vi "IMAQ FPGA Camera Link Pixel Packer U16x1.vi"(8 "Input Valid":bool, 9 "Frame Valid In":bool, 10 "Line Valid In":bool, 11 "Pixel In":u16) -> (0 "Output Valid":bool, 1 "Frame Valid Out":bool, 2 "Line Valid Out":bool, 3 "Pixel Bus x8 Out":cluster{"Pixels":u16[], "DV":bool[]})   [LabVIEW 2020]
doc: "The Pixel Packer combines pixels from different cycles to create a Pixel Bus with 8 adjacent pixels. The DV flag in the Pixel Bus x8 Out indicates if the corresponding pixel is valid in case there are cameras with a width that is not a multiple of 8."
uses:
  <vilib>/visionFPGA/Basics/Camera Link Acquisition/Controls/IMAQ FPGA Camera Link Pixel Packer State.ctl
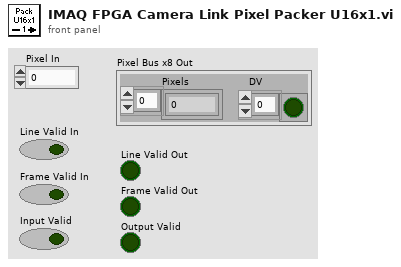
[diagram p1: front panel]
types:
  T1 = typedef "IMAQ FPGA Camera Link Pixel Packer State.ctl" = enum16{"Wait to Pack", "Pack", "Add EOL", "Check EOI"}
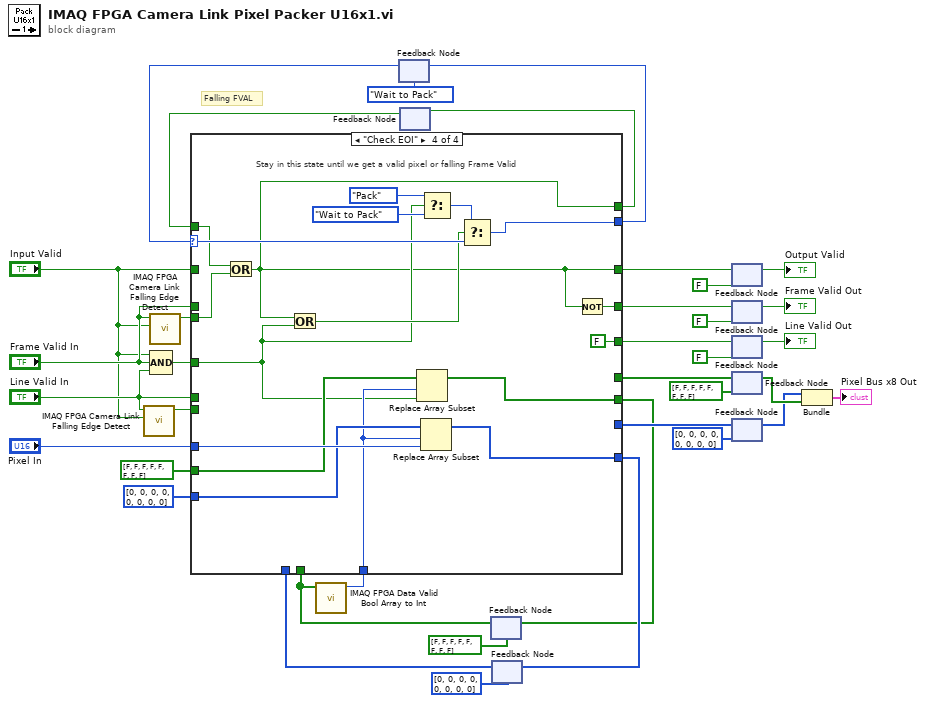
[diagram p0: block diagram]
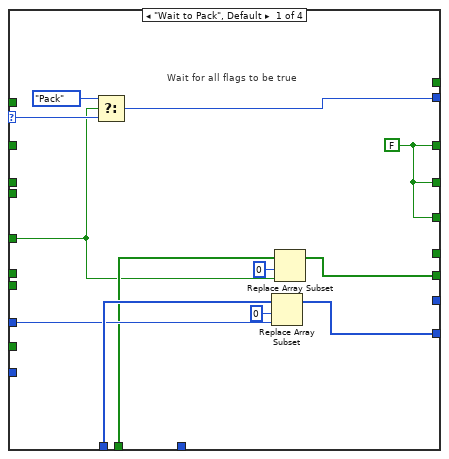
[diagram p2: hidden frame]
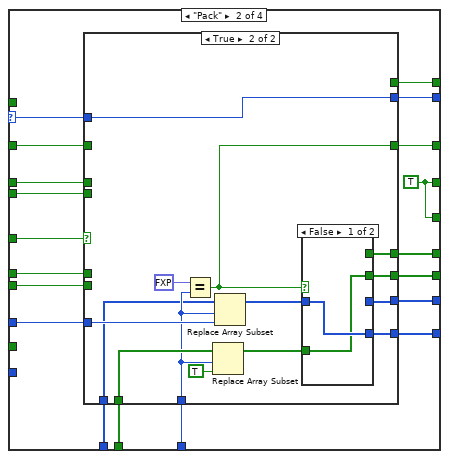
[diagram p3: hidden frame]
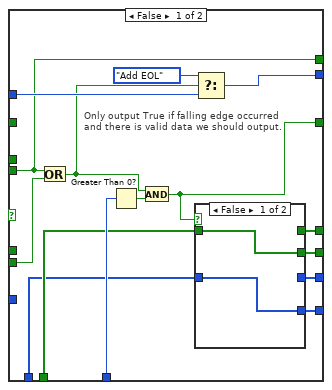
[diagram p4: hidden frame]
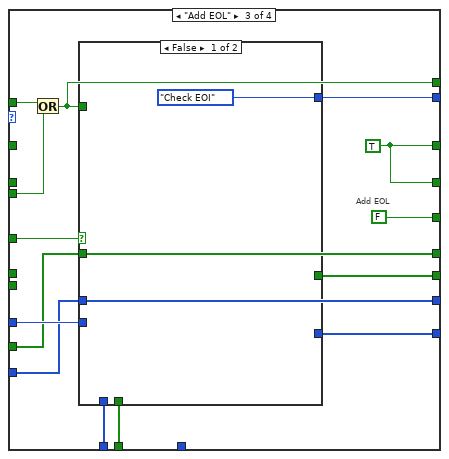
[diagram p7: hidden frame]
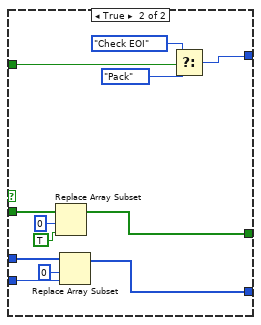
[diagram p8: hidden frame]
diagram:
  # "Falling FVAL"
  n1 = call <vilib>:"IMAQ FPGA Camera Link Falling Edge Detect.vi"("Input Valid"="Input Valid", "Input"="Line Valid In") -> ("Falling Edge"=w7:bool)  [unwired: 9 in]
  n2 = call <vilib>:"IMAQ FPGA Camera Link Falling Edge Detect.vi"("Input Valid"="Input Valid", "Input"="Frame Valid In") -> ("Falling Edge"=w10:bool)  [unwired: 9 in]
  n3 = Compound Arithmetic op=AND("Input Valid", "Frame Valid In", "Line Valid In") -> (w16:bool)
  n4 = feedback #1(IMAQ_FPGA_Camera_Link_Pixel_Packer_State."Wait to Pack" ("Enum")) -> (w18:T1)
  n5 = feedback #2() -> (w3:bool)  [unwired: 1 in]
  n6 = feedback #3(bool[] [FALSE, FALSE, FALSE, FALSE, FALSE, FALSE, FALSE, FALSE]) -> (w2:bool[])
  n7 = call <vilib>:"IMAQ FPGA Data Valid Bool Array to Int.vi"("DV In"=w2) -> ("Sum DV Out"=w1:u8)  [unwired: 10 in]
  n8 = feedback #4(u16[] [0, 0, 0, 0, 0, 0, 0, 0] ("Pixels")) -> (w30:u16[])
  n9 = case shown="\"Check EOI\"" w18 {
    selector: w18 -> [w49 w67 _ w150]
    tunnel: w2 -> [w43 w55 w115 _]
    tunnel: w30 -> [w47 w66 w116 _]
    tunnel: [_ w63 w109 _] -> w29
    tunnel: [_ w62 w110 _] -> w22
    tunnel: [w38 w61 w119 w134] -> w36
    tunnel: [w38 w52 w119 w133] -> w20
    tunnel: [w38 w52 FALSE FALSE ("Frame Valid In")] -> w19
    tunnel: "Frame Valid In" -> [_ w59 _ _]
    tunnel: "Line Valid In" -> [_ w60 _ _]
    tunnel: "Input Valid" -> [_ w58 _ _]
    tunnel: w16 -> [w40 w68 w118 w136]
    tunnel: "Pixel In" -> [w45 w56 w113 w145]
    tunnel: [w44 w65 w112 w143] -> w14
    tunnel: [w41 w64 w114 w144] -> w13
    tunnel: [w39 w57 w117 w149] -> w12
    tunnel: w10 -> [_ w54 w107 w138]
    tunnel: w7 -> [_ w53 _ _]
    tunnel: bool[] [FALSE, FALSE, FALSE, FALSE, FALSE, FALSE, FALSE, FALSE] -> [_ _ w110 w142]
    tunnel: u16[] [0, 0, 0, 0, 0, 0, 0, 0] ("Pixels") -> [_ _ w109 w141]
    tunnel: [_ w51 w106 w134] -> w4
    tunnel: w3 -> [_ _ w108 w137]
    tunnel: w1 -> [_ w50 _ w139]
    frame "Wait to Pack", Default {
      w38 = FALSE
      # "Wait for all flags to be true"
      n10 = Select(t=IMAQ_FPGA_Camera_Link_Pixel_Packer_State."Pack", s=w40, f=w49) -> (s? t:f=w39:T1)
      n11 = Replace Array Subset(array=w47, new element=w45, index=0) -> (w44:u16[])
      n12 = Replace Array Subset(array=w43, new element=w40, index=0) -> (w41:bool[])
    }
    frame "Pack" {
      w52 = TRUE ("Frame Valid In")
      n13 = case shown="True" w68 {
        tunnel: w67 -> [w82 w99]
        tunnel: [w80 w99] -> w57
        tunnel: w66 -> [w73 w92]
        tunnel: [w78 w89] -> w65
        tunnel: w55 -> [w74 w101]
        tunnel: [w77 w95] -> w64
        tunnel: [w71 w90] -> w63
        tunnel: [w72 w96] -> w62
        tunnel: w58 -> [_ _]
        tunnel: [w70 w98] -> w61
        tunnel: w59 -> [_ _]
        tunnel: w60 -> [_ _]
        tunnel: w54 -> [w69 _]
        tunnel: w53 -> [w83 _]
        tunnel: w50 -> [w79 w93]
        tunnel: w56 -> [_ w94]
        tunnel: [w69 _] -> w51
        frame False {
          # "Only output True if falling edge occurred and there is valid data we should output."
          n14 = Or(x=w69, y=w83) -> (x .or. y?=w75:bool)
          n15 = Greater Than 0?(x=w79) -> (x > 0?=w76:bool)
          n16 = And(x=w75, y=w76) -> (x .and. y?=w70:bool)
          n17 = case shown="False" w70 {
            tunnel: [w84 _] -> w78
            tunnel: [w85 _] -> w77
            tunnel: w74 -> [w85 w87]
            tunnel: w73 -> [w84 w86]
            tunnel: [_ w87] -> w72
            tunnel: [_ w86] -> w71
            frame False {
            }
            frame True {
            }
          }
          n18 = Select(t=IMAQ_FPGA_Camera_Link_Pixel_Packer_State."Add EOL", s=w75, f=w82) -> (s? t:f=w80:T1)
        }
        frame True {
          n19 = Equal?(x=fxp<+,4,4> 7.0, y=w93) -> (x = y?=w98:bool)
          n20 = Replace Array Subset(array=w101, new element=TRUE ("new element/subarray"), index=w93) -> (w97:bool[])
          n21 = Replace Array Subset(array=w92, new element=w94, index=w93) -> (w91:u16[])
          n22 = case shown="False" w98 {
            tunnel: w97 -> [w102 w105]
            tunnel: [_ w105] -> w96
            tunnel: [w102 _] -> w95
            tunnel: w91 -> [w103 w104]
            tunnel: [_ w104] -> w90
            tunnel: [w103 _] -> w89
            frame False {
            }
            frame True {
            }
          }
        }
      }
    }
    frame "Add EOL" {
      w119 = TRUE
      # "Add EOL"
      n23 = Or(x=w108, y=w107) -> (x .or. y?=w106:bool)
      n24 = case shown="False" w118 {
        tunnel: [IMAQ_FPGA_Camera_Link_Pixel_Packer_State."Check EOI" ("Enum") w121] -> w117
        tunnel: w116 -> [_ _]
        tunnel: w115 -> [_ _]
        tunnel: w110 -> [_ w132]
        tunnel: [_ w130] -> w114
        tunnel: w109 -> [_ w128]
        tunnel: w113 -> [_ w127]
        tunnel: [_ w125] -> w112
        tunnel: w106 -> [_ w124]
        frame False {
        }
        frame True {
          n25 = Replace Array Subset(array=w132, new element=TRUE ("new element/subarray"), index=0) -> (w130:bool[])
          n26 = Replace Array Subset(array=w128, new element=w127, index=0) -> (w125:u16[])
          n27 = Select(t=IMAQ_FPGA_Camera_Link_Pixel_Packer_State."Check EOI" ("Enum"), s=w124, f=IMAQ_FPGA_Camera_Link_Pixel_Packer_State."Pack" ("Enum")) -> (s? t:f=w121:T1)
        }
      }
    }
    frame "Check EOI" {
      # "Stay in this state until we get a valid pixel or falling Frame Valid"
      n28 = Or(x=w137, y=w138) -> (x .or. y?=w134:bool)
      n29 = Or(x=w134, y=w136) -> (x .or. y?=w140:bool)
      n30 = Replace Array Subset(array=w142, new element=w136, index=w139) -> (w144:bool[])
      n31 = Replace Array Subset(array=w141, new element=w145, index=w139) -> (w143:u16[])
      n32 = Select(t=IMAQ_FPGA_Camera_Link_Pixel_Packer_State."Pack" ("Enum"), s=w136, f=IMAQ_FPGA_Camera_Link_Pixel_Packer_State."Wait to Pack" ("Enum")) -> (s? t:f=w146:T1)
      n33 = Select(t=w146, s=w140, f=w150) -> (s? t:f=w149:T1)
      n34 = Not(x=w134) -> (.not. x?=w133:bool)
    }
  }
  n35 = feedback-in #1(w12) -> ()
  n36 = feedback-in #2(w4) -> ()
  n37 = feedback-in #3(w13) -> ()
  n38 = feedback-in #4(w14) -> ()
  n39 = feedback #5(FALSE) -> (→"Output Valid":bool)
  n40 = feedback-in #5(w36) -> ()
  n41 = feedback #6(FALSE) -> (→"Frame Valid Out":bool)
  n42 = feedback-in #6(w20) -> ()
  n43 = feedback #7(FALSE) -> (→"Line Valid Out":bool)
  n44 = feedback-in #7(w19) -> ()
  n45 = feedback #8(bool[] [FALSE, FALSE, FALSE, FALSE, FALSE, FALSE, FALSE, FALSE]) -> (w27:bool[])
  n46 = feedback-in #8(w22) -> ()
  n47 = feedback #9(u16[] [0, 0, 0, 0, 0, 0, 0, 0] ("Pixels")) -> (w26:u16[])
  n48 = feedback-in #9(w29) -> ()
  n49 = Bundle("Pixels"=w26, w27) -> (→"Pixel Bus x8 Out":cluster{"Pixels":u16[], bool[]})  [unwired: 1 in]
